vi "Default Instrument Setup.vi"(8 "error in (no error)":errorcluster, 11 "VISA resource name":refnum<visa-resource-name>) -> (0 "error out":errorcluster, 3 "VISA resource name out":refnum<visa-resource-name>)   [LabVIEW 2025, in "NewtonsPSM1735.lvlib"]
doc: "This Utility VI sends a default command string to the instrument ."
uses:
  NewtonsPSM1735.lvlib
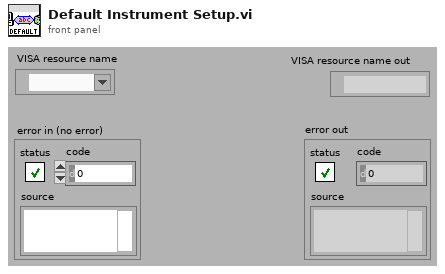
[diagram p1: front panel]
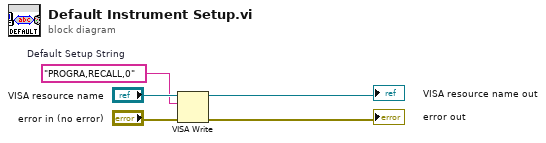
[diagram p0: block diagram]
diagram:
  w3 = "PROGRA,RECALL,0"  # Default Setup String
  n1 = VISA Write(VISA resource name="VISA resource name", write buffer=w3, error in (no error)="error in (no error)") -> (VISA resource name out=→"VISA resource name out":refnum<visa-resource-name>, error out=→"error out":errorcluster)  [unwired: 1 out]
